vi "SWM.vi"(8 "Stopp":bool, 10 "SLOT":i32=100 min=0 max=999 step=100 format="%03d", 11 "USB":i32) -> ()   [LabVIEW 2020]
doc: "This VI provides a GUI for SWM modules. It implements an abstract module interface, where callers provide the only necessary and sufficient information for callee modules via the datafields USB, SLOT and Stopp. All module intern information are handled hidden by the module. Thereby, a caller must not \"know\" about such internals."
panel:
  out "CrvPar2":T1
  out "CrvPar1":T1
  in  "ExtAtten":sgl caption="Ext. Atten. [dB]" min=-99 max=0 step=3 format="%.1f"
  in  "SlewRate2":sgl caption="Pulse Start [ns]" min=0 max=20 step=0.02 format="%.3f"
  in  "SlewRate1":sgl caption="Slew Rate   [V/µs]" min=0 max=20 step=0.02 format="%.3f"
  in  "PulseAmp2":sgl caption="Pulse Start [ns]" min=0 max=1 step=0.001 format="%.3f"
  in  "PulseAmp1":sgl caption="Amplitude    [V]" min=0 max=1 step=0.001 format="%.3f"
  in  "CurveStop2":sgl caption="Pulse Start [ns]" min=0 max=330 step=0.33 format="%.3f"
  in  "CurveStop1":sgl caption="Curve Stop [ns]" min=0 max=330 step=0.33 format="%.3f"
  in  "RampStart2":sgl caption="Pulse Start [ns]" min=0 max=330 step=0.33 format="%.3f"
  in  "RampStart1":sgl caption="Ramp Start [ns]" min=0 max=330 step=0.33 format="%.3f"
  in  "PulseStart2":sgl caption="Pulse Start [ns]" min=0 max=330 step=0.33 format="%.3f"
  in  "PulseStart1":sgl caption="Pulse Start  [ns]" min=0 max=330 step=0.33 format="%.3f"
  in  "TimeBase2":u16(ring) caption="Time Base" items=["33 ns", "100 ns", "330 ns"]
  in  "TimeBase1":u16(ring) caption="Time Base" items=["33 ns", "100 ns", "330 ns"]
  out "TB_UpperLimits":i32[](array[numeric])
  # "Curve 1    |    Curve 2"
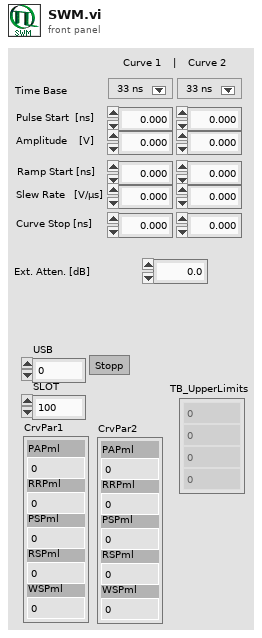
[diagram p1: front panel]
types:
  T1 = cluster{"PAPml":u16, "RRPml":u16, "PSPml":u16, "RSPml":u16, "WSPml":u16}
  T2 = cluster{"TBNdx":u8, "PAPml":u16, "RRPml":u16, "PSPml":u16, "RSPml":u16, "WSPml":u16}
  T3 = cluster{"TBNdxCount":u8, "MaxAmplitude":u16, "MaxSlewRate":u16, "ExpRampEffect":u16, "MinUserValue":u16, "MaxUserValue":u16, "UserResolution":u16}
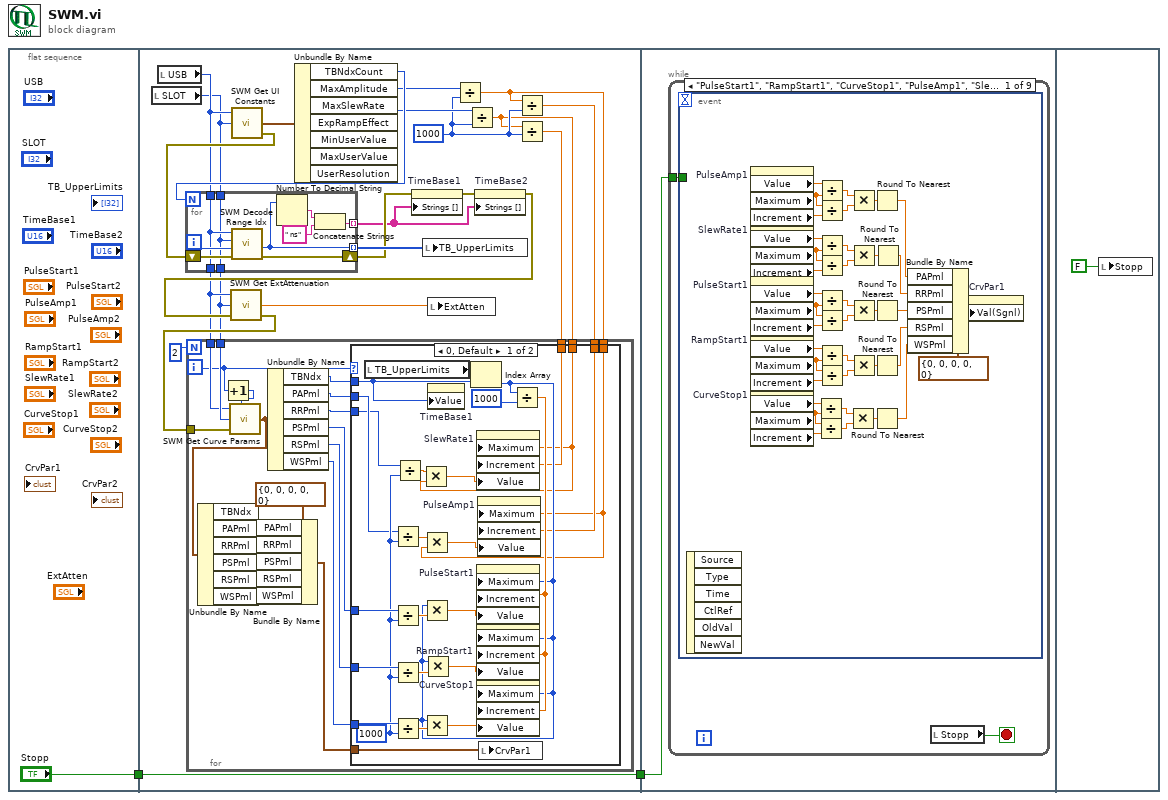
[diagram p0: block diagram]
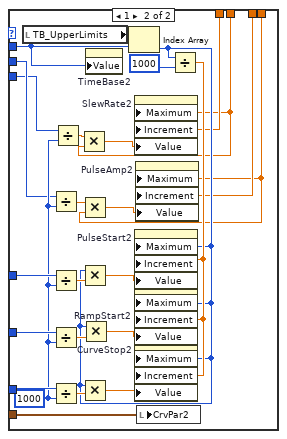
[diagram p2: hidden frame]
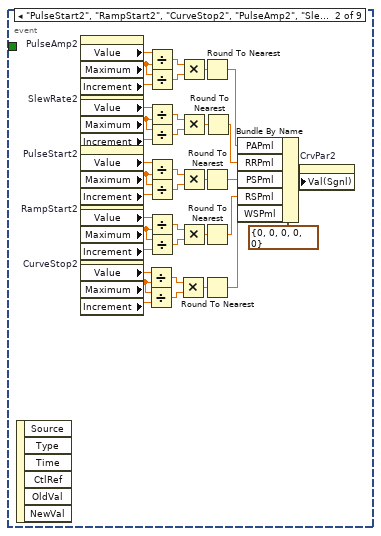
[diagram p3: hidden frame]
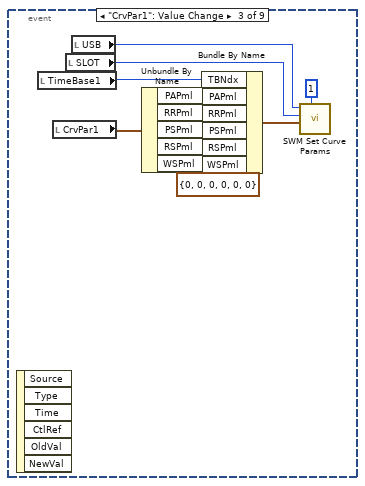
[diagram p4: hidden frame]
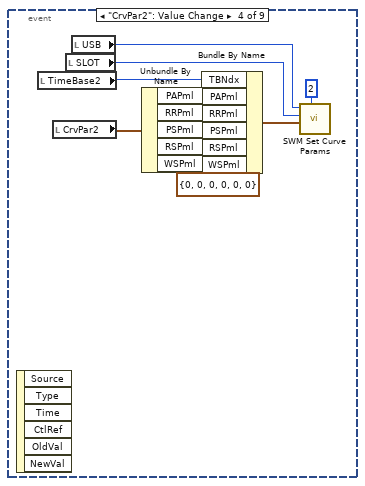
[diagram p5: hidden frame]
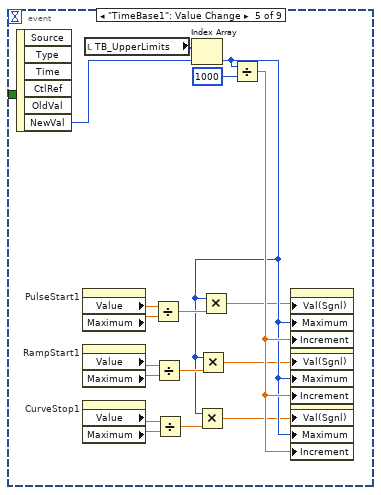
[diagram p6: hidden frame]
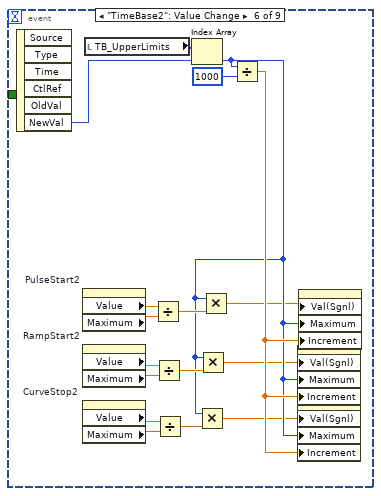
[diagram p7: hidden frame]
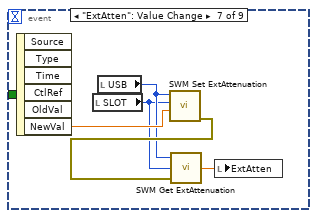
[diagram p8: hidden frame]
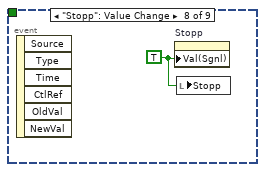
[diagram p9: hidden frame]
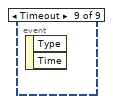
[diagram p10: hidden frame]
diagram:
  n1 = flat-sequence {
    tunnel: ["Stopp"] -> w1
    tunnel: [w17] -> w2
    tunnel: w1 -> [w17]
    tunnel: w2 -> [w111]
    frame #0 {
    }
    frame #1 {
      w12 = 1000
      n2 = local read "SLOT"() -> (w22:i32)
      n3 = local read "USB"() -> (w23:i32)
      n4 = call "SWM Get UI Constants.vi"("SlotId"=w22, "DevIdx"=w23) -> ("error out"=w24:errorcluster, "SWM UI Constants"=w26:T3)  [unwired: 1 in, 1 out]
      n5 = Unbundle By Name(w26) -> ("TBNdxCount"=w25:u8, "MaxAmplitude"=w15:u16, "MaxSlewRate"=w14:u16)  [unwired: 4 out]
      n6 = for {
        N: w25 -> [_]
        tunnel: w23 -> [w107]
        shift-right: [w108] -> w19
        shift-left: w24 -> [w110]
        tunnel: w22 -> [w106]
        tunnel: [w107] -> w5
        tunnel: [w106] -> w4
        tunnel: [w102] -> w21 mode=indexing
        tunnel: [w103] -> w18 mode=indexing
        i -> [w109]
        n7 = call "SWM Decode Range Idx.vi"("error in (no error)"=w110, "RangeIdx"=w109, "SlotId"=w106, "DevIdx"=w107) -> ("error out"=w108:errorcluster, "UpperLimit"=w102:i32)  [unwired: 1 in, 1 out]
        n8 = Number To Decimal String(number=w102) -> (decimal integer string=w105:string)  [unwired: 1 in]
        n9 = Concatenate Strings(w105, " ns" ("string")) -> (w103:string)
      }
      n10 = property on="TimeBase1" class="Ring (strict)"(error in=w19, "Strings []"=w18) -> (error out=w20:errorcluster)  [unwired: 1 in, 1 out]
      n11 = local write "TB_UpperLimits"(w21) -> ()
      n12 = Divide(x=w15, y=w12) -> (x/y=w13:dbl)
      n13 = Divide(x=w14, y=w12) -> (x/y=w11:dbl)
      n14 = property on="TimeBase2" class="Ring (strict)"(error in=w20, "Strings []"=w18) -> (error out=w8:errorcluster)  [unwired: 1 in, 1 out]
      n15 = call "SWM Get ExtAttenuation.vi"("error in (no error)"=w8, "SlotId"=w4, "DevIdx"=w5) -> ("error out"=w7:errorcluster, "ExtAtt"=w6:sgl)  [unwired: 1 out]
      n16 = local write "ExtAtten"(w6) -> ()
      n17 = Divide(x=w13, y=w12) -> (x/y=w10:dbl)
      n18 = Divide(x=w11, y=w12) -> (x/y=w9:dbl)
      n19 = for {
        N: 2 ("CurveIdx") -> [_]
        tunnel: w7 -> [w49]
        tunnel: w4 -> [w47]
        tunnel: w5 -> [w46]
        tunnel: w13 -> [w37]
        tunnel: w11 -> [w38]
        tunnel: w10 -> [w36]
        tunnel: w9 -> [w39]
        i -> [w45]
        n20 = Increment(x=w45) -> (x+1=w48:i32)
        n21 = call "SWM Get Curve Params.vi"("DevIdx"=w46, "CurveIdx"=w48, "SlotId"=w47, "error in (no error)"=w49) -> ("SWM Curve Params"=w34:T2)  [unwired: 1 in, 2 out]
        n22 = Unbundle By Name(w34) -> ("PAPml"=w33:u16, "RRPml"=w32:u16, "PSPml"=w31:u16, "RSPml"=w30:u16, "WSPml"=w29:u16)  [unwired: 1 out]
        n23 = Bundle By Name(cluster=T1 {"PAPml"=0, "RRPml"=0, "PSPml"=0, "RSPml"=0, "WSPml"=0} ("SWM Curve Params"), "PAPml"=w33, "RRPml"=w32, "PSPml"=w31, "RSPml"=w30, "WSPml"=w29) -> (w27:T1)
        n24 = Unbundle By Name(w34) -> ("TBNdx"=w44:u8, "PAPml"=w35:u16, "RRPml"=w40:u16, "PSPml"=w41:u16, "RSPml"=w42:u16, "WSPml"=w43:u16)
        n25 = case shown="0, Default" w45 {
          tunnel: w44 -> [w74 w100]
          tunnel: w35 -> [w58 w84]
          tunnel: w43 -> [w71 w97]
          tunnel: w42 -> [w70 w96]
          tunnel: w41 -> [w69 w95]
          tunnel: w40 -> [w57 w83]
          tunnel: w39 -> [w60 w86]
          tunnel: w38 -> [w52 w78]
          tunnel: w37 -> [w51 w77]
          tunnel: w36 -> [w59 w85]
          tunnel: w27 -> [w50 w76]
          frame 0, Default {
            w61 = 1000
            n26 = local read "TB_UpperLimits"() -> (w75:i32[])
            n27 = Divide(x=w58, y=w61) -> (x/y=w54:dbl)
            n28 = Divide(x=w69, y=w61) -> (x/y=w68:dbl)
            n29 = Divide(x=w70, y=w61) -> (x/y=w66:dbl)
            n30 = Divide(x=w71, y=w61) -> (x/y=w67:dbl)
            n31 = Divide(x=w57, y=w61) -> (x/y=w55:dbl)
            n32 = Multiply(x=w55, y=w52) -> (x*y=w53:dbl)
            n33 = Multiply(x=w54, y=w51) -> (x*y=w56:dbl)
            n34 = property on="TimeBase1" class="Ring (strict)"("Value"=w74) -> ()  [unwired: 2 in, 2 out]
            n35 = Index Array(array=w75, index=w74) -> (element=w65:i32)
            n36 = Multiply(x=w65, y=w68) -> (x*y=w62:dbl)
            n37 = Multiply(x=w65, y=w67) -> (x*y=w64:dbl)
            n38 = Multiply(x=w65, y=w66) -> (x*y=w63:dbl)
            n39 = property on="SlewRate1" class="DigNum (strict)"("Maximum"=w52, "Increment"=w60, "Value"=w53) -> ()  [unwired: 2 in, 2 out]
            n40 = property on="PulseAmp1" class="DigNum (strict)"("Maximum"=w51, "Increment"=w59, "Value"=w56) -> ()  [unwired: 2 in, 2 out]
            n41 = local write "CrvPar1"(w50) -> ()
            n42 = Divide(x=w65, y=1000) -> (x/y=w72:dbl)
            n43 = property on="PulseStart1" class="DigNum (strict)"("Maximum"=w65, "Increment"=w72, "Value"=w62) -> ()  [unwired: 2 in, 2 out]
            n44 = property on="RampStart1" class="DigNum (strict)"("Maximum"=w65, "Increment"=w72, "Value"=w63) -> ()  [unwired: 2 in, 2 out]
            n45 = property on="CurveStop1" class="DigNum (strict)"("Maximum"=w65, "Increment"=w72, "Value"=w64) -> ()  [unwired: 2 in, 2 out]
          }
          frame 1 {
            w87 = 1000
            n46 = local read "TB_UpperLimits"() -> (w101:i32[])
            n47 = Divide(x=w84, y=w87) -> (x/y=w80:dbl)
            n48 = Divide(x=w95, y=w87) -> (x/y=w94:dbl)
            n49 = Divide(x=w96, y=w87) -> (x/y=w92:dbl)
            n50 = Divide(x=w97, y=w87) -> (x/y=w93:dbl)
            n51 = Divide(x=w83, y=w87) -> (x/y=w81:dbl)
            n52 = Multiply(x=w81, y=w78) -> (x*y=w79:dbl)
            n53 = Multiply(x=w80, y=w77) -> (x*y=w82:dbl)
            n54 = property on="TimeBase2" class="Ring (strict)"("Value"=w100) -> ()  [unwired: 2 in, 2 out]
            n55 = Index Array(array=w101, index=w100) -> (element=w91:i32)
            n56 = Multiply(x=w91, y=w94) -> (x*y=w88:dbl)
            n57 = Multiply(x=w91, y=w93) -> (x*y=w90:dbl)
            n58 = Multiply(x=w91, y=w92) -> (x*y=w89:dbl)
            n59 = property on="SlewRate2" class="DigNum (strict)"("Maximum"=w78, "Increment"=w86, "Value"=w79) -> ()  [unwired: 2 in, 2 out]
            n60 = property on="PulseAmp2" class="DigNum (strict)"("Maximum"=w77, "Increment"=w85, "Value"=w82) -> ()  [unwired: 2 in, 2 out]
            n61 = local write "CrvPar2"(w76) -> ()
            n62 = Divide(x=w91, y=1000) -> (x/y=w98:dbl)
            n63 = property on="PulseStart2" class="DigNum (strict)"("Maximum"=w91, "Increment"=w98, "Value"=w88) -> ()  [unwired: 2 in, 2 out]
            n64 = property on="RampStart2" class="DigNum (strict)"("Maximum"=w91, "Increment"=w98, "Value"=w89) -> ()  [unwired: 2 in, 2 out]
            n65 = property on="CurveStop2" class="DigNum (strict)"("Maximum"=w91, "Increment"=w98, "Value"=w90) -> ()  [unwired: 2 in, 2 out]
          }
        }
      }
    }
    frame #2 {
      n66 = while {
        tunnel: w111 -> [w112]
        stop <- w113 stop-if-true
        n67 = event shown="[0] \"PulseStart1\", \"RampStart1\", \"CurveStop1\", \"PulseAmp1\", \"SlewRate1\": Value Change" {
          selector: _ -> [_ _ _ _ _ _ _ _ _]
          dyn-events: _ -> [_ _ _ _ _ _ _ _ _]
          timeout: _ -> [_ _ _ _ _ _ _ _ _]
          tunnel: w112 -> [_ _ _ _ _ _ _ _ _]
          event "PulseStart1", "RampStart1", "CurveStop1", "PulseAmp1", "SlewRate1": Value Change {
            n68 = event-data() -> ()  [unwired: 1 in, 6 out]
            n69 = property on="PulseAmp1" class="DigNum (strict)"() -> ("Value"=w133:sgl, "Maximum"=w132:dbl, "Increment"=w131:dbl)  [unwired: 2 in, 2 out]
            n70 = property on="SlewRate1" class="DigNum (strict)"() -> ("Value"=w128:sgl, "Maximum"=w127:dbl, "Increment"=w126:dbl)  [unwired: 2 in, 2 out]
            n71 = property on="PulseStart1" class="DigNum (strict)"() -> ("Value"=w150:sgl, "Maximum"=w149:dbl, "Increment"=w148:dbl)  [unwired: 2 in, 2 out]
            n72 = property on="RampStart1" class="DigNum (strict)"() -> ("Value"=w143:sgl, "Maximum"=w142:dbl, "Increment"=w141:dbl)  [unwired: 2 in, 2 out]
            n73 = property on="CurveStop1" class="DigNum (strict)"() -> ("Value"=w138:sgl, "Maximum"=w137:dbl, "Increment"=w136:dbl)  [unwired: 2 in, 2 out]
            n74 = Divide(x=w138, y=w137) -> (x/y=w134:dbl)
            n75 = Divide(x=w137, y=w136) -> (x/y=w135:dbl)
            n76 = Divide(x=w133, y=w132) -> (x/y=w129:dbl)
            n77 = Divide(x=w132, y=w131) -> (x/y=w130:dbl)
            n78 = Divide(x=w128, y=w127) -> (x/y=w124:dbl)
            n79 = Divide(x=w127, y=w126) -> (x/y=w125:dbl)
            n80 = Divide(x=w150, y=w149) -> (x/y=w146:dbl)
            n81 = Divide(x=w149, y=w148) -> (x/y=w147:dbl)
            n82 = Divide(x=w143, y=w142) -> (x/y=w139:dbl)
            n83 = Divide(x=w142, y=w141) -> (x/y=w140:dbl)
            n84 = Multiply(x=w134, y=w135) -> (x*y=w122:dbl)
            n85 = Multiply(x=w129, y=w130) -> (x*y=w123:dbl)
            n86 = Multiply(x=w124, y=w125) -> (x*y=w119:dbl)
            n87 = Multiply(x=w146, y=w147) -> (x*y=w120:dbl)
            n88 = Multiply(x=w139, y=w140) -> (x*y=w121:dbl)
            n89 = Round To Nearest(number=w123) -> (nearest integer value=w118:dbl)
            n90 = Round To Nearest(number=w120) -> (nearest integer value=w114:dbl)
            n91 = Round To Nearest(number=w121) -> (nearest integer value=w116:dbl)
            n92 = Round To Nearest(number=w122) -> (nearest integer value=w117:dbl)
            n93 = Round To Nearest(number=w119) -> (nearest integer value=w115:dbl)
            n94 = Bundle By Name(cluster=T1 {"PAPml"=0, "RRPml"=0, "PSPml"=0, "RSPml"=0, "WSPml"=0} ("CrvPar1"), "PAPml"=w118, "RRPml"=w115, "PSPml"=w114, "RSPml"=w116, "WSPml"=w117) -> (w144:T1)
            n95 = property on="CrvPar1" class="Clust (strict)"("Val(Sgnl)"=w144) -> ()  [unwired: 2 in, 2 out]
          }
          event "PulseStart2", "RampStart2", "CurveStop2", "PulseAmp2", "SlewRate2": Value Change {
            n96 = event-data() -> ()  [unwired: 1 in, 6 out]
            n97 = property on="PulseAmp2" class="DigNum (strict)"() -> ("Value"=w170:sgl, "Maximum"=w169:dbl, "Increment"=w168:dbl)  [unwired: 2 in, 2 out]
            n98 = property on="SlewRate2" class="DigNum (strict)"() -> ("Value"=w165:sgl, "Maximum"=w164:dbl, "Increment"=w163:dbl)  [unwired: 2 in, 2 out]
            n99 = property on="PulseStart2" class="DigNum (strict)"() -> ("Value"=w187:sgl, "Maximum"=w186:dbl, "Increment"=w185:dbl)  [unwired: 2 in, 2 out]
            n100 = property on="RampStart2" class="DigNum (strict)"() -> ("Value"=w180:sgl, "Maximum"=w179:dbl, "Increment"=w178:dbl)  [unwired: 2 in, 2 out]
            n101 = property on="CurveStop2" class="DigNum (strict)"() -> ("Value"=w175:sgl, "Maximum"=w174:dbl, "Increment"=w173:dbl)  [unwired: 2 in, 2 out]
            n102 = Divide(x=w175, y=w174) -> (x/y=w171:dbl)
            n103 = Divide(x=w174, y=w173) -> (x/y=w172:dbl)
            n104 = Divide(x=w170, y=w169) -> (x/y=w166:dbl)
            n105 = Divide(x=w169, y=w168) -> (x/y=w167:dbl)
            n106 = Divide(x=w165, y=w164) -> (x/y=w161:dbl)
            n107 = Divide(x=w164, y=w163) -> (x/y=w162:dbl)
            n108 = Divide(x=w187, y=w186) -> (x/y=w183:dbl)
            n109 = Divide(x=w186, y=w185) -> (x/y=w184:dbl)
            n110 = Divide(x=w180, y=w179) -> (x/y=w176:dbl)
            n111 = Divide(x=w179, y=w178) -> (x/y=w177:dbl)
            n112 = Multiply(x=w171, y=w172) -> (x*y=w159:dbl)
            n113 = Multiply(x=w166, y=w167) -> (x*y=w160:dbl)
            n114 = Multiply(x=w161, y=w162) -> (x*y=w156:dbl)
            n115 = Multiply(x=w183, y=w184) -> (x*y=w157:dbl)
            n116 = Multiply(x=w176, y=w177) -> (x*y=w158:dbl)
            n117 = Round To Nearest(number=w160) -> (nearest integer value=w155:dbl)
            n118 = Round To Nearest(number=w157) -> (nearest integer value=w151:dbl)
            n119 = Round To Nearest(number=w158) -> (nearest integer value=w153:dbl)
            n120 = Round To Nearest(number=w159) -> (nearest integer value=w154:dbl)
            n121 = Round To Nearest(number=w156) -> (nearest integer value=w152:dbl)
            n122 = Bundle By Name(cluster=T1 {"PAPml"=0, "RRPml"=0, "PSPml"=0, "RSPml"=0, "WSPml"=0} ("CrvPar1"), "PAPml"=w155, "RRPml"=w152, "PSPml"=w151, "RSPml"=w153, "WSPml"=w154) -> (w181:T1)
            n123 = property on="CrvPar2" class="Clust (strict)"("Val(Sgnl)"=w181) -> ()  [unwired: 2 in, 2 out]
          }
          event "CrvPar1": Value Change {
            n124 = event-data() -> ()  [unwired: 1 in, 6 out]
            n125 = local read "TimeBase1"() -> (w194:u16)
            n126 = local read "CrvPar1"() -> (w193:T1)
            n127 = local read "SLOT"() -> (w195:i32)
            n128 = local read "USB"() -> (w196:i32)
            n129 = Unbundle By Name(w193) -> ("PAPml"=w192:u16, "RRPml"=w191:u16, "PSPml"=w190:u16, "RSPml"=w189:u16, "WSPml"=w188:u16)
            n130 = Bundle By Name(cluster=T2 {"TBNdx"=0, "PAPml"=0, "RRPml"=0, "PSPml"=0, "RSPml"=0, "WSPml"=0} ("SWM Curve Params"), "TBNdx"=w194, "PAPml"=w192, "RRPml"=w191, "PSPml"=w190, "RSPml"=w189, "WSPml"=w188) -> (w197:T2)
            n131 = call "SWM Set Curve Params.vi"("DevIdx"=w196, "SlotId"=w195, "SWM Curve Params"=w197, "CurveIdx"=1) -> ()  [unwired: 1 in, 2 out]
          }
          event "CrvPar2": Value Change {
            n132 = event-data() -> ()  [unwired: 1 in, 6 out]
            n133 = local read "TimeBase2"() -> (w206:u16)
            n134 = local read "CrvPar2"() -> (w205:T1)
            n135 = local read "SLOT"() -> (w207:i32)
            n136 = local read "USB"() -> (w208:i32)
            n137 = Unbundle By Name(w205) -> ("PAPml"=w204:u16, "RRPml"=w203:u16, "PSPml"=w202:u16, "RSPml"=w201:u16, "WSPml"=w200:u16)
            n138 = Bundle By Name(cluster=T2 {"TBNdx"=0, "PAPml"=0, "RRPml"=0, "PSPml"=0, "RSPml"=0, "WSPml"=0} ("SWM Curve Params"), "TBNdx"=w206, "PAPml"=w204, "RRPml"=w203, "PSPml"=w202, "RSPml"=w201, "WSPml"=w200) -> (w209:T2)
            n139 = call "SWM Set Curve Params.vi"("DevIdx"=w208, "SlotId"=w207, "SWM Curve Params"=w209, "CurveIdx"=2) -> ()  [unwired: 1 in, 2 out]
          }
          event "TimeBase1": Value Change {
            n140 = event-data() -> ("NewVal"=w220:u16)  [unwired: 1 in, 5 out]
            n141 = property on="PulseStart1" class="DigNum (strict)"() -> ("Value"=w227:sgl, "Maximum"=w228:dbl)  [unwired: 2 in, 2 out]
            n142 = property on="RampStart1" class="DigNum (strict)"() -> ("Value"=w226:sgl, "Maximum"=w225:dbl)  [unwired: 2 in, 2 out]
            n143 = property on="CurveStop1" class="DigNum (strict)"() -> ("Value"=w223:sgl, "Maximum"=w224:dbl)  [unwired: 2 in, 2 out]
            n144 = local read "TB_UpperLimits"() -> (w222:i32[])
            n145 = Divide(x=w227, y=w228) -> (x/y=w216:dbl)
            n146 = Divide(x=w226, y=w225) -> (x/y=w217:dbl)
            n147 = Divide(x=w223, y=w224) -> (x/y=w218:dbl)
            n148 = Index Array(array=w222, index=w220) -> (element=w215:i32)
            n149 = Multiply(x=w215, y=w218) -> (x*y=w212:dbl)
            n150 = Multiply(x=w215, y=w217) -> (x*y=w213:dbl)
            n151 = Multiply(x=w215, y=w216) -> (x*y=w214:dbl)
            n152 = Divide(x=w215, y=1000) -> (x/y=w219:dbl)
            n153 = property on="PulseStart1" class="DigNum (strict)"("Val(Sgnl)"=w214, "Maximum"=w215, "Increment"=w219) -> ()  [unwired: 2 in, 2 out]
            n154 = property on="RampStart1" class="DigNum (strict)"("Val(Sgnl)"=w213, "Maximum"=w215, "Increment"=w219) -> ()  [unwired: 2 in, 2 out]
            n155 = property on="CurveStop1" class="DigNum (strict)"("Val(Sgnl)"=w212, "Maximum"=w215, "Increment"=w219) -> ()  [unwired: 2 in, 2 out]
          }
          event "TimeBase2": Value Change {
            n156 = event-data() -> ("NewVal"=w237:u16)  [unwired: 1 in, 5 out]
            n157 = property on="PulseStart2" class="DigNum (strict)"() -> ("Value"=w244:sgl, "Maximum"=w245:dbl)  [unwired: 2 in, 2 out]
            n158 = property on="RampStart2" class="DigNum (strict)"() -> ("Value"=w243:sgl, "Maximum"=w242:dbl)  [unwired: 2 in, 2 out]
            n159 = property on="CurveStop2" class="DigNum (strict)"() -> ("Value"=w240:sgl, "Maximum"=w241:dbl)  [unwired: 2 in, 2 out]
            n160 = local read "TB_UpperLimits"() -> (w239:i32[])
            n161 = Divide(x=w244, y=w245) -> (x/y=w233:dbl)
            n162 = Divide(x=w243, y=w242) -> (x/y=w234:dbl)
            n163 = Divide(x=w240, y=w241) -> (x/y=w235:dbl)
            n164 = Index Array(array=w239, index=w237) -> (element=w232:i32)
            n165 = Multiply(x=w232, y=w235) -> (x*y=w229:dbl)
            n166 = Multiply(x=w232, y=w234) -> (x*y=w230:dbl)
            n167 = Multiply(x=w232, y=w233) -> (x*y=w231:dbl)
            n168 = Divide(x=w232, y=1000) -> (x/y=w236:dbl)
            n169 = property on="RampStart2" class="DigNum (strict)"("Val(Sgnl)"=w230, "Maximum"=w232, "Increment"=w236) -> ()  [unwired: 2 in, 2 out]
            n170 = property on="CurveStop2" class="DigNum (strict)"("Val(Sgnl)"=w229, "Maximum"=w232, "Increment"=w236) -> ()  [unwired: 2 in, 2 out]
            n171 = property on="PulseStart2" class="DigNum (strict)"("Val(Sgnl)"=w231, "Maximum"=w232, "Increment"=w236) -> ()  [unwired: 2 in, 2 out]
          }
          event "ExtAtten": Value Change {
            n172 = event-data() -> ("NewVal"=w250:sgl)  [unwired: 1 in, 5 out]
            n173 = local read "SLOT"() -> (w247:i32)
            n174 = local read "USB"() -> (w248:i32)
            n175 = call "SWM Set ExtAttenuation.vi"("ExtAtt"=w250, "SlotId"=w247, "DevIdx"=w248) -> ("error out"=w249:errorcluster)  [unwired: 3 in, 1 out]
            n176 = call "SWM Get ExtAttenuation.vi"("error in (no error)"=w249, "SlotId"=w247, "DevIdx"=w248) -> ("ExtAtt"=w246:sgl)  [unwired: 2 out]
            n177 = local write "ExtAtten"(w246) -> ()
          }
          event "Stopp": Value Change {
            w251 = TRUE ("Value (Signaling)")
            n178 = event-data() -> ()  [unwired: 1 in, 6 out]
            n179 = property on="Stopp" class="Bool (strict)"("Val(Sgnl)"=w251) -> ()  [unwired: 2 in, 2 out]
            n180 = local write "Stopp"(w251) -> ()
          }
          event Timeout {
            n181 = event-data() -> ()  [unwired: 1 in, 2 out]
          }
        }
        n182 = local read "Stopp"() -> (w113:bool)
      }
    }
    frame #3 {
      n183 = local write "Stopp"(FALSE ("Stopp")) -> ()
    }
  }
